vi "pulse Tx.vi"(9 "enable line":bool=TRUE, 10 "take it!":bool, 11 "Cluster":T1={"PW"=0, "frequency shift"=0.0, "amp"=0.9999923706054688, "mode type"=enum."CW", "mode depth"=0, "mode filter"=0, "phase shift"=0.0, "pulse shape filter"=0}) -> (1 "output valid":bool, 2 "data out":T3, 3 "free dds":bool, 4 "frequncy":fxp<+/-,48,0>, 6 "phase":fxp<+/-,16,1>)   [LabVIEW 2021]
uses:
  <instrlib>/_niInstr/DSP/v1/Shared/Public/IQ Data.ctl
  pulse_tx_vis/pdw.ctl
  pulse_tx_vis/CTL/mode_type.ctl
  <instrlib>/_niInstr/Basic Elements/v1/FPGA/Private/Count Up U32.vi
  <instrlib>/_niInstr/DSP/v1/FPGA/Public/Sub VIs/Frequency Shift/Frequency Shift - 1 spc.vi
  <vilib>/rvi/FXPMathLib/FxpAdd/XNode/nifxpmath_Add.xnode
  <instrlib>/_niInstr/DSP/v1/XNodes/Public/Frequency Shift/niInstr DSP v1 Frequency Shift FPGA.xnode
  <instrlib>/_niInstr/DSP/v1/Shared/niInstr DSP v1 Shared.lvlib
  <instrlib>/_niInstr/Basic Elements/v1/FPGA/niInstr Basic Elements v1 FPGA.lvlib
  <vilib>/rvi/FXPMathLib/sim/FxpSim.dll
  <instrlib>/_niInstr/DSP/v1/FPGA/niInstr DSP v1 FPGA.lvlib
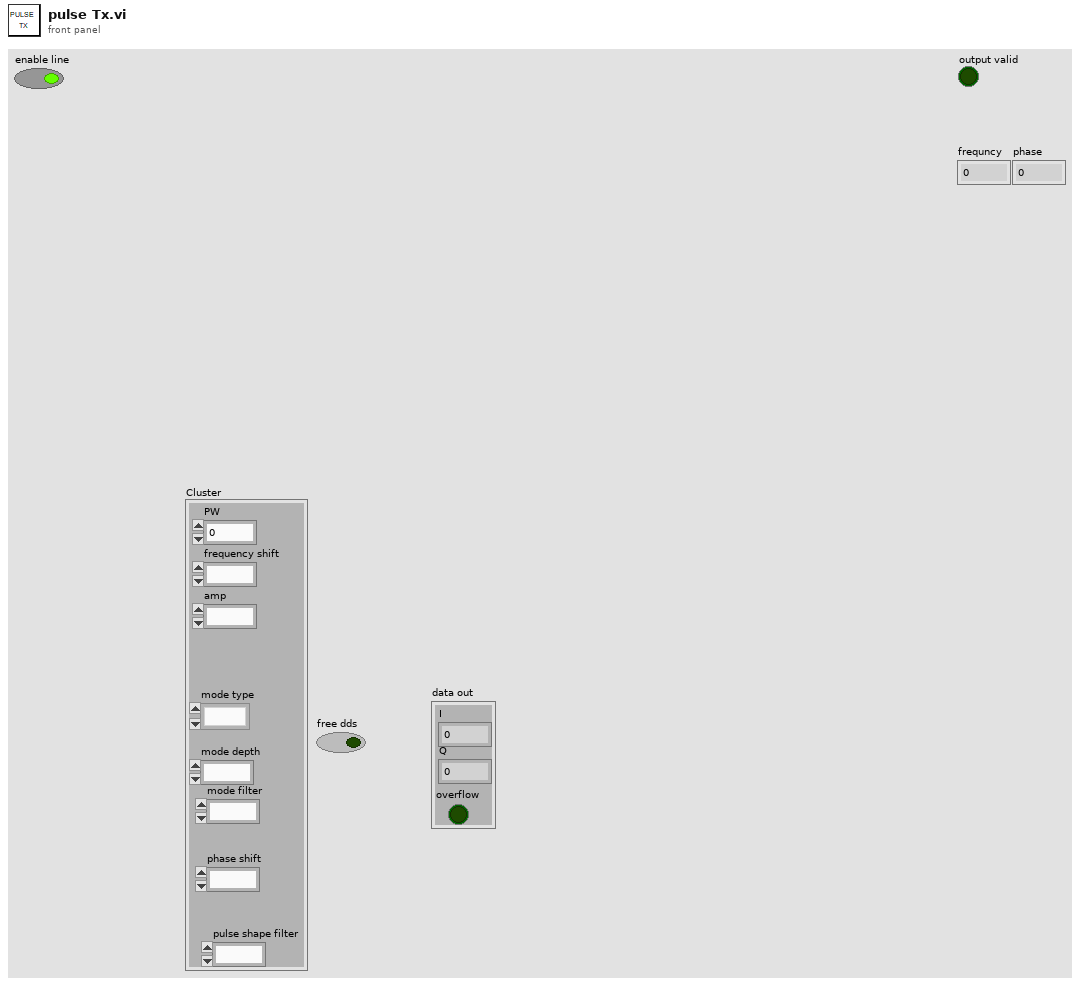
[diagram p1: front panel]
types:
  T1 = typedef "pdw.ctl" = cluster{"PW":u32, "frequency shift":fxp<+/-,48,0>, "amp":fxp<+/-,18,1>, "mode type":T2, "mode depth":u32, "mode filter":u8, "phase shift":fxp<+/-,16,1>, "pulse shape filter":u8}
  T2 = typedef "mode_type.ctl" = enum8{"CW", "NC - CW", "NC - cw", "LFM", "BPSK", "QPSK"}
  T3 = typedef "niInstr DSP v1 Shared.lvlib/IQ Data.ctl" = cluster{"I":fxp<+/-,18,1>, "Q":fxp<+/-,18,1>, "overflow":bool}
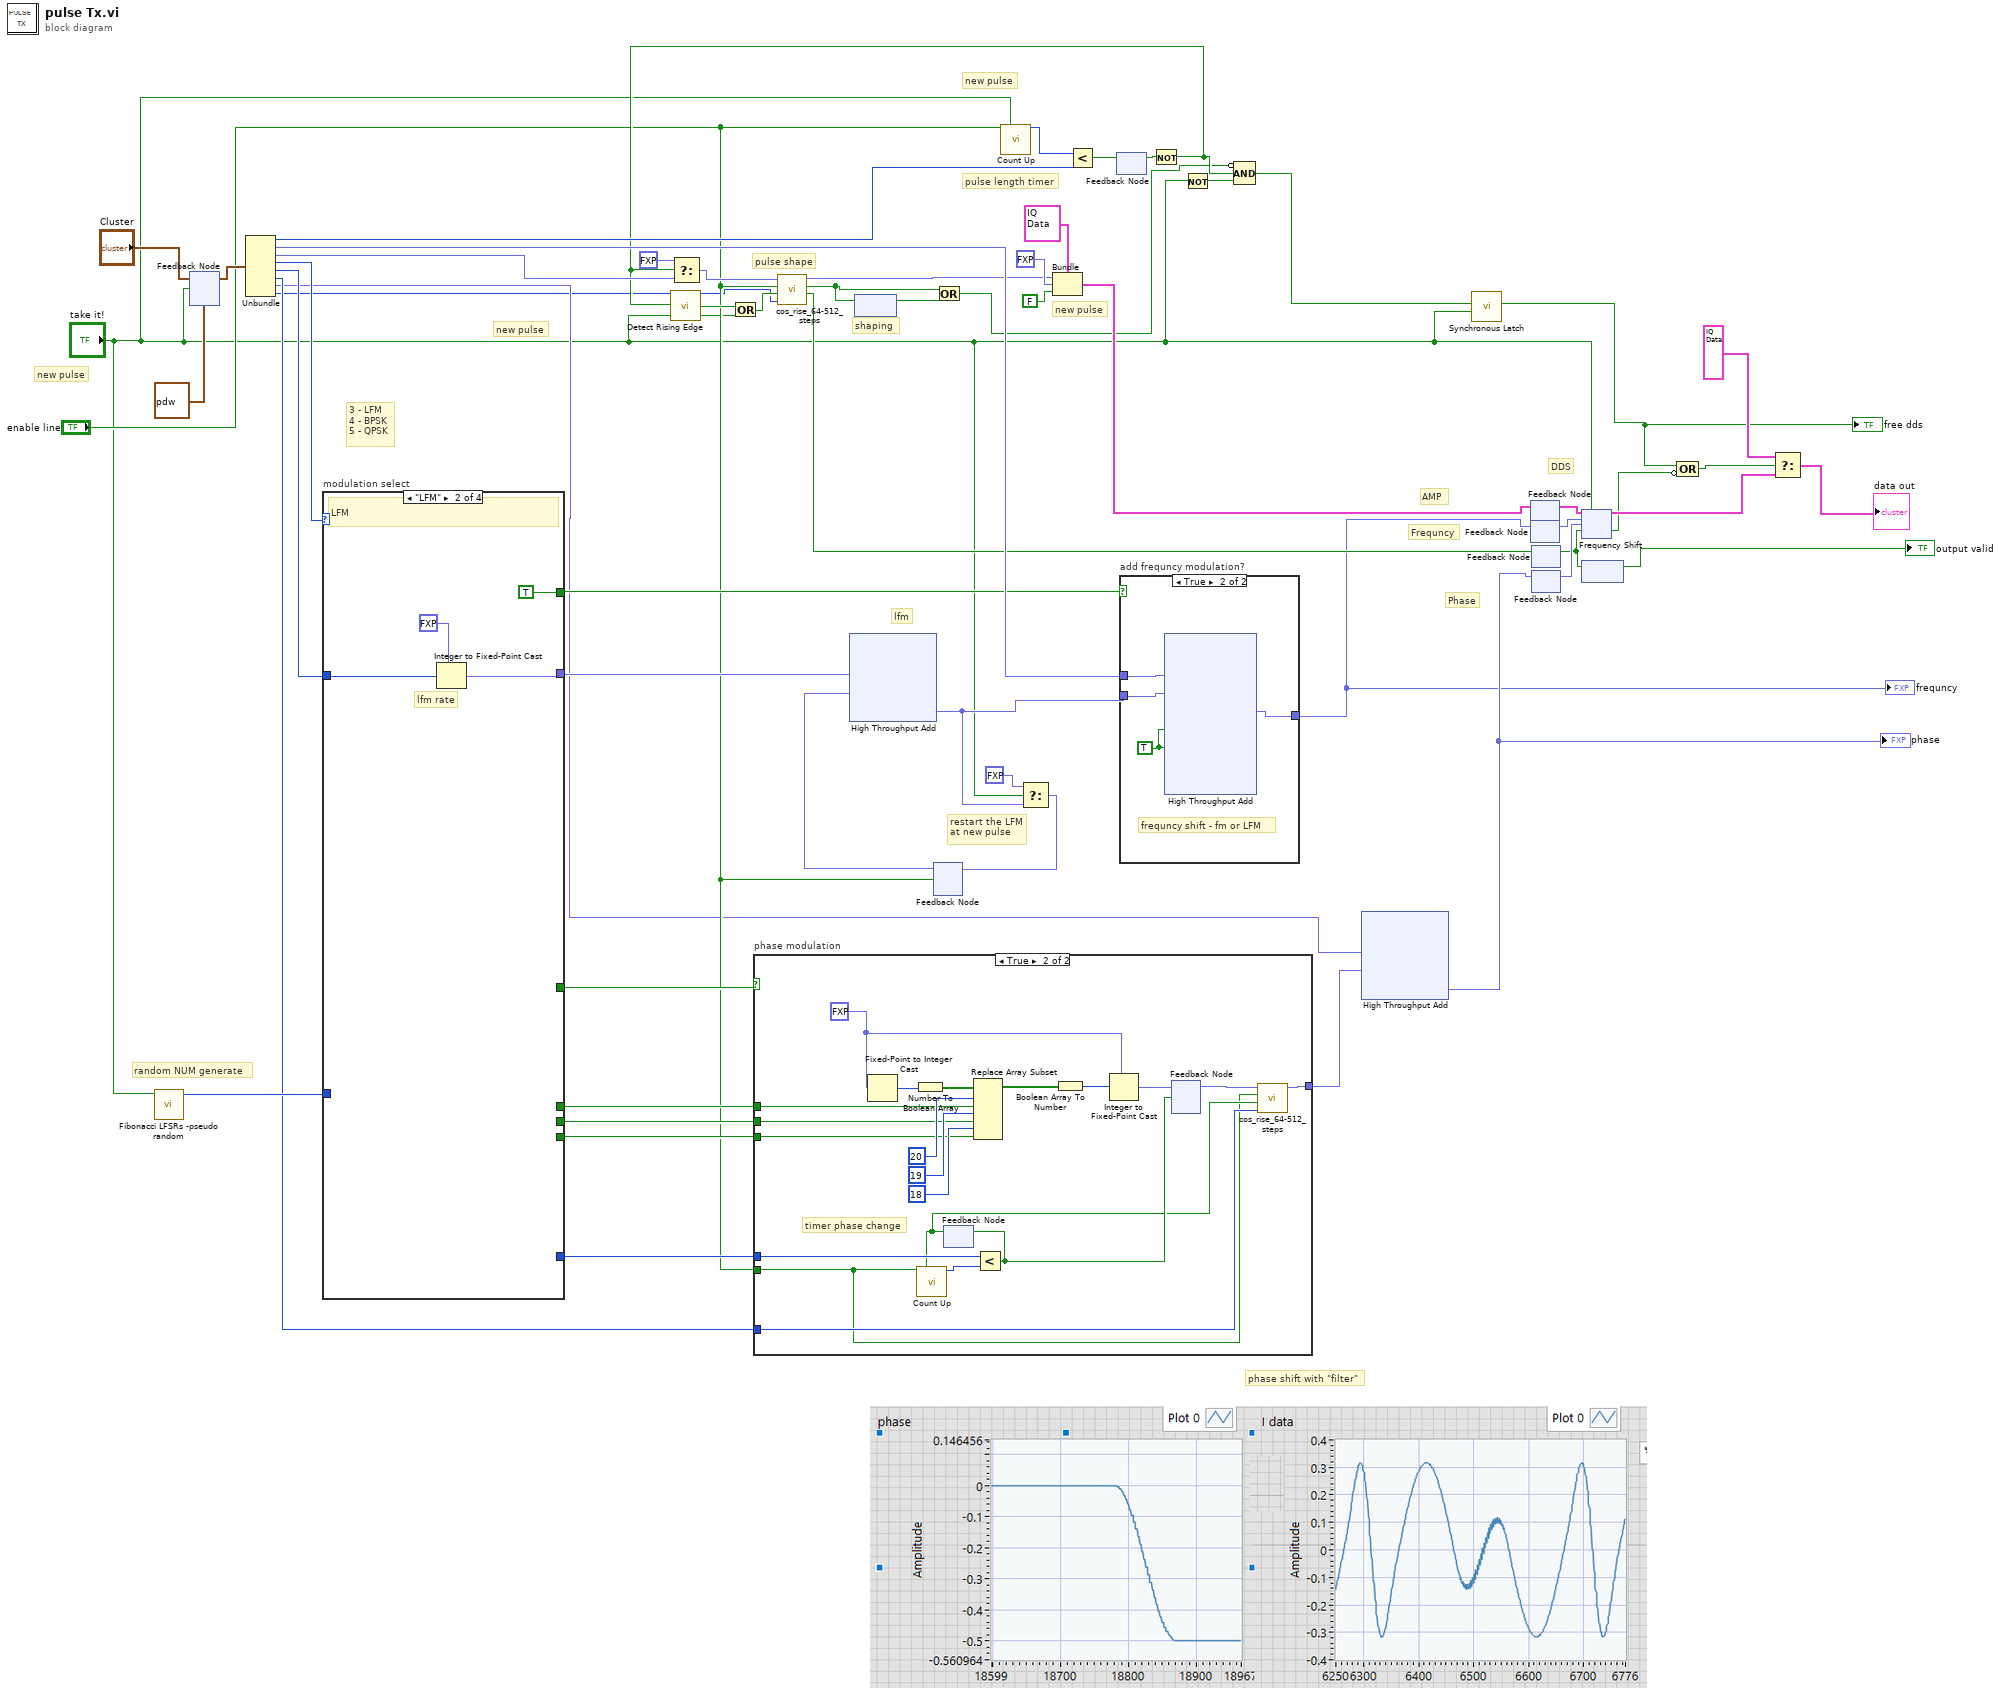
[diagram p0: block diagram]
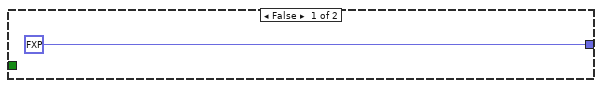
[diagram p2: hidden frame]
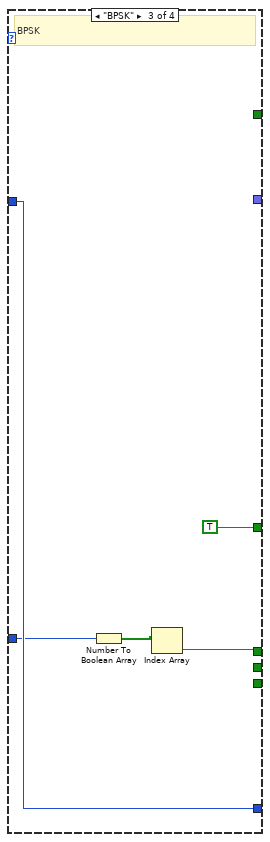
[diagram p5: hidden frame]
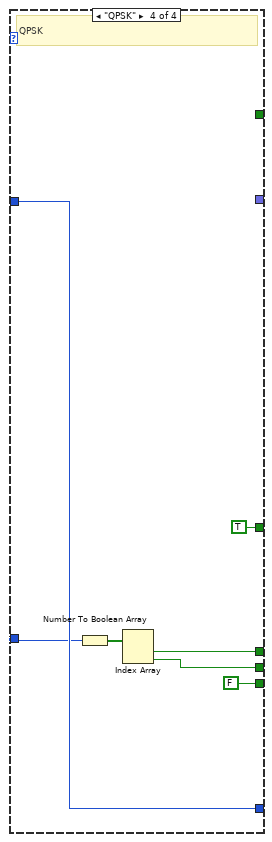
[diagram p6: hidden frame]
diagram:
  # "random NUM generate"
  # "phase shift with \"filter\""
  # "Phase"
  # "Frequncy"
  # "AMP"
  # "DDS"
  # "shaping"
  # "3 - LFM\n4 - BPSK\n5 - QPSK"
  # "pulse length timer"
  # "restart the LFM\nat new pulse"
  # "lfm"
  # "pulse shape"
  # "new pulse"
  # "new pulse"
  # "new pulse"
  # "new pulse"
  n1 = call "Fibonacci LFSRs -pseudo random.vi"("reset random"="take it!") -> ("rand number"=w30:u16)  [unwired: 10 in]
  n2 = feedback #1(T1 {"PW"=0, "frequency shift"=0.0, "amp"=0.9999923706054688, "mode type"=enum."CW", "mode depth"=0, "mode filter"=0, "phase shift"=0.0, "pulse shape filter"=0} ("Cluster")) -> (w54:T1)
  n3 = feedback-in #1("Cluster", "take it!") -> ()
  n4 = Unbundle(w54) -> ("PW"=w58:u32, "frequency shift"=w50:fxp<+/-,48,0>, "amp"=w33:fxp<+/-,18,1>, "mode type"=w51:T2, "mode depth"=w25:u32, "mode filter"=w24:u8, "phase shift"=w19:fxp<+/-,16,1>, "pulse shape filter"=w9:u8)
  n5 = case "modulation select" shown="\"LFM\"" w51 {
    tunnel: w25 -> [_ w61 w64 w69]
    tunnel: [_ w60 _ _] -> w46
    tunnel: [_ TRUE ("s") _ _] -> w43
    tunnel: [_ _ _ FALSE] -> w41
    tunnel: [_ _ _ w71] -> w40
    tunnel: [_ _ w66 w73] -> w39
    tunnel: [_ _ TRUE TRUE] -> w38
    tunnel: [_ _ w64 w69] -> w37
    tunnel: w30 -> [_ _ w63 w68]
    frame Default {
    }
    frame "LFM" {
      # "lfm rate"
      # "LFM"
      n6 = Integer to Fixed-Point Cast(fixed-point type=fxp<+,32,-16> 0.0, integer=w61) -> (fixed-point=w60:fxp<+,32,-16>)
    }
    frame "BPSK" {
      # "BPSK"
      n7 = Number To Boolean Array(number=w63) -> (Boolean array=w67:bool[])
      n8 = Index Array(array=w67) -> (element=w66:bool)  [unwired: 1 in]
    }
    frame "QPSK" {
      # "QPSK"
      n9 = Number To Boolean Array(number=w68) -> (Boolean array=w74:bool[])
      n10 = Index Array(array=w74) -> (element #1=w73:bool, element #2=w71:bool)  [unwired: 2 in]
    }
  }
  n11 = case "phase modulation" shown="True" w38 {
    tunnel: w41 -> [_ w87]
    tunnel: w40 -> [_ w86]
    tunnel: w39 -> [_ w85]
    tunnel: w37 -> [_ w83]
    tunnel: [fxp<+/-,16,1> 0.0 ("filter out") w79] -> w18
    tunnel: w24 -> [_ w77]
    tunnel: "enable line" -> [_ w76]
    frame False {
    }
    frame True {
      w89 = fxp<+/-,21,0> 0.0 ("phase")
      # "timer phase change"
      n12 = Fixed-Point to Integer Cast(1:w89) -> (0:w95:i32)
      n13 = Number To Boolean Array(number=w95) -> (Boolean array=w93:bool[])
      n14 = feedback #2() -> (w78:bool)  [unwired: 1 in]
      n15 = call-poly <instrlib>:"Count Up.vi"("increment"=w76, "reset"=w78) -> ("count out"=w82:u32)  [unwired: 13 in]
      n16 = Replace Array Subset(array=w93, new element #1=w85, index #1=20 ("index"), new element #2=w86, index #2=19 ("index"), new element #3=w87, index #3=18 ("index")) -> (w88:bool[])
      n17 = Less?(x=w83, y=w82) -> (x < y?=w81:bool)
      n18 = feedback-in #2(w81) -> ()
      n19 = Boolean Array To Number(Boolean array=w88) -> (number=w94:u32)
      n20 = Integer to Fixed-Point Cast(fixed-point type=w89, integer=w94) -> (fixed-point=w84:fxp<+/-,21,0>)
      n21 = feedback-in #3(w84, w81) -> ()
      n22 = feedback #3() -> (w80:fxp<+/-,21,0>)  [unwired: 1 in]
      n23 = call "cos_rise_64-512_steps.vi"("filter select"=w77, "new step"=w78, "run"=w76, "data in"=w80) -> ("data out"=w79:fxp<+/-,16,1>)  [unwired: 5 in, 2 out]
    }
  }
  n24 = feedback #4() -> (w2:bool)  [unwired: 1 in]
  n25 = feedback #5() -> (w45:fxp<+/-,48,0>)  [unwired: 1 in]
  n26 = xnode ("High Throughput Add")("x"=w46, "y"=w45) -> ("x+y"=w44:fxp<+/-,48,0>)
  n27 = call-poly <instrlib>:"Count Up.vi"("increment"="enable line", "reset"="take it!") -> ("count out"=w36:u32)  [unwired: 13 in]
  n28 = Select(t=fxp<+/-,48,0> 0.0, s="take it!", f=w44) -> (s? t:f=w47:fxp<+/-,48,0>)
  n29 = feedback-in #5(w47, "enable line") -> ()
  n30 = Less?(x=w36, y=w58) -> (x < y?=w35:bool)
  n31 = feedback #6() -> (w34:bool)  [unwired: 1 in]
  n32 = feedback-in #6(w35) -> ()
  n33 = case "add frequncy modulation?" shown="True" w43 {
    tunnel: w50 -> [w96 w100]
    tunnel: w44 -> [_ w99]
    tunnel: [w96 w98] -> w15
    frame False {
    }
    frame True {
      w97 = TRUE ("input valid")
      # "frequncy shift - fm or LFM"
      n34 = xnode ("High Throughput Add")("x"=w100, "y"=w99, "input valid"=w97, "ready for output (T)"=w97) -> ("x+y"=w98:fxp<+/-,48,0>)  [unwired: 2 out]
    }
  }
  "frequncy" <- w15
  n35 = Not(x=w34) -> (.not. x?=w27:bool)
  n36 = call <instrlib>:"Detect Rising Edge.vi"("signal"=w27) -> ("edge detected"=w26:bool)  [unwired: 14 in]
  n37 = Select(t=fxp<+/-,18,1> 0.0, s=w27, f=w33) -> (s? t:f=w32:fxp<+/-,18,1>)
  n38 = Or(x=w26, y="take it!") -> (x .or. y?=w28:bool)
  n39 = call "cos_rise_64-512_steps.vi"("filter select"=w9, "new step"=w28, "run"="enable line", "data in"=w32) -> ("output valid"=w16:bool, "steping"=w3:bool, "data out"=w29:fxp<+/-,16,1>)  [unwired: 5 in]
  n40 = feedback-in #4(w3) -> ()
  n41 = Or(x=w3, y=w2) -> (x .or. y?=w1:bool)
  n42 = Bundle(cluster=T3 {"I"=0.9999923706054688, "Q"=0.0, "overflow"=FALSE} ("data"), "I"=w29, "Q"=fxp<+/-,18,1> 0.0, "overflow"=FALSE ("input valid")) -> (w14:T3)
  n43 = Not(x="take it!") -> (.not. x?=w53:bool)
  n44 = Compound Arithmetic op=AND(invert w1, w27, w53) -> (w52:bool)
  n45 = xnode ("High Throughput Add")("x"=w19, "y"=w18) -> ("x+y"=w17:fxp<+/-,16,1>)
  "phase" <- w17
  n46 = call <instrlib>:"Synchronous Latch.vi"("clear"="take it!", "set"=w52) -> ("out"=w8:bool)  [unwired: 9 in]
  "free dds" <- w8
  n47 = feedback #7() -> (w11:T3)  [unwired: 1 in]
  n48 = feedback-in #7(w14) -> ()
  n49 = feedback #8() -> (w12:fxp<+/-,48,0>)  [unwired: 1 in]
  n50 = feedback-in #8(w15) -> ()
  n51 = feedback #9() -> (w5:bool)  [unwired: 1 in]
  n52 = feedback-in #9(w16) -> ()
  n53 = feedback-in #10(w17) -> ()
  n54 = feedback #10() -> (w13:fxp<+/-,16,1>)  [unwired: 1 in]
  n55 = xnode "Frequency Shift"("data in"=w11, "reset"="take it!", "frequency shift"=w12, "phase"=w13, "input valid"=w5) -> ("data out"=w22:T3, "output valid"=w6:bool)  [unwired: 1 in, 1 out]
  n56 = feedback #11() -> (→"output valid":bool)  [unwired: 1 in]
  n57 = feedback-in #11(w5) -> ()
  n58 = Compound Arithmetic op=OR(w8, invert w6) -> (w7:bool)
  n59 = Select(t=T3 {"I"=0.0, "Q"=0.0, "overflow"=FALSE}, s=w7, f=w22) -> (s? t:f=→"data out":T3)
